vi "Tremolo.vi"(2 "error in":errorcluster, 3 "frequency":dbl=0.0078125 format="%0.4e", 4 "amplitude":dbl=1.0 format="%0.2f", 5 "samples":dbl=128.0) -> (0 "error out":errorcluster, 1 "signal out":dbl[](array[numeric]))   [LabVIEW 2019]
uses:
  <vilib>/Analysis/NI_AALBase.lvlib
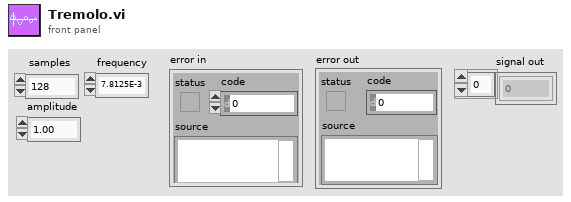
[diagram p1: front panel]
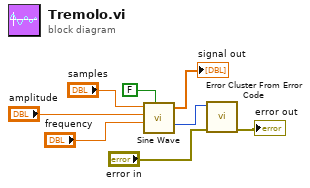
[diagram p0: block diagram]
diagram:
  n1 = call <vilib>:"Sine Wave.vi"("samples"="samples", "amplitude"="amplitude", "frequency"="frequency", "reset phase"=FALSE) -> ("sine wave"=→"signal out":dbl[], "error"=w4:i32)  [unwired: 1 in, 1 out]
  n2 = call <vilib>:"Error Cluster From Error Code.vi"("error in (no error)"="error in", "error code (0)"=w4) -> ("error out"=→"error out":errorcluster)  [unwired: 7 in]
